vi "Configure Transform Precoding.vi"(6 "Enabled (On)":bool=TRUE, 7 "Bandwidth Part (BWP0)":T1 items=["BWP0"], 8 "error in (no error)":errorcluster, 9 "Carrier Component (1)":T2=1, 10 "Instance (1)":T3=1, 11 "VISA resource name":refnum<visa-resource-name>) -> (0 "error out":errorcluster, 3 "VISA resource name out":refnum<visa-resource-name>)   [LabVIEW 2020, in "Rohde&Schwarz CMXP NR FR2 Measurement.lvlib"]
doc: "Specifies whether the <BWP> on carrier <no> uses a transform precoding function.\n\nAttribute:\nRSCMXPNRFR2M_ATTR_TRANSFORM_PRECODING\n\nRemote-control command:\nCONFigure:NRMMw:MEAS<i>[:CC<no>]:BWPart:PUSCh:DFTPrecoding"
uses:
  <instrlib>/Rohde&Schwarz CMXP NR FR2 Measurement/Rohde&Schwarz CMXP NR FR2 Measurement.lvlib
  <instrlib>/Rohde&Schwarz CMXP NR FR2 Measurement/Private/_Instance.ctl
  <instrlib>/Rohde&Schwarz CMXP NR FR2 Measurement/Private/_Carrier Component.ctl
  <instrlib>/Rohde&Schwarz CMXP NR FR2 Measurement/Private/_Bandwidth Part.ctl
  <instrlib>/Rohde&Schwarz CMXP NR FR2 Measurement/Private/rsidr_core.llb/rsidr_core.lvlib
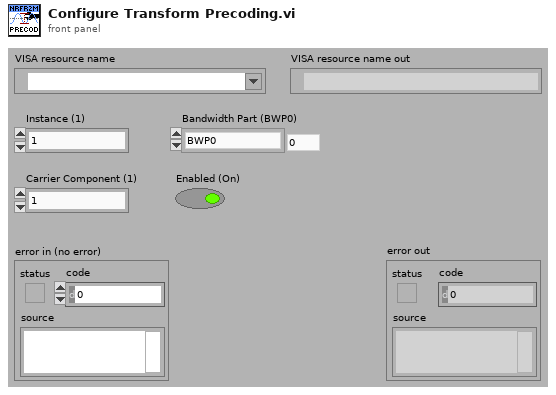
[diagram p1: front panel]
types:
  T1 = typedef "Rohde&Schwarz CMXP NR FR2 Measurement.lvlib/_Bandwidth Part.ctl" = i32
  T2 = typedef "Rohde&Schwarz CMXP NR FR2 Measurement.lvlib/_Carrier Component.ctl" = i32
  T3 = typedef "Rohde&Schwarz CMXP NR FR2 Measurement.lvlib/_Instance.ctl" = i32
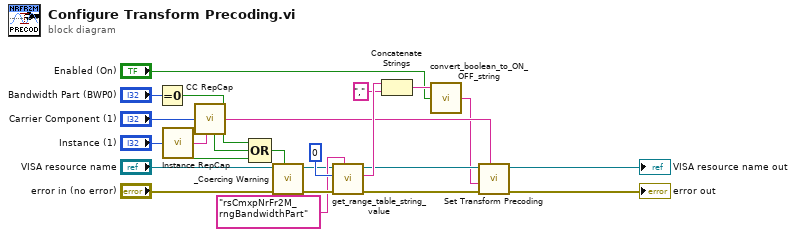
[diagram p0: block diagram]
diagram:
  n1 = Equal To 0?(x="Bandwidth Part (BWP0)") -> (x = 0?=w4:bool)
  n2 = call <instrlib>:"Instance RepCap.vi"("Instance In"="Instance (1)") -> ("In Range?"=w20:bool, "RepCap Identifier Out"=w2:string)  [unwired: 1 in]
  n3 = call <instrlib>:"CC RepCap.vi"("CC In"="Carrier Component (1)", "RepCap String In (\"\")"=w2) -> ("In Range?"=w19:bool, "RepCap Identifier Out"=w11:string)
  n4 = Compound Arithmetic op=OR(w4, w19, w20) -> (w21:bool)
  n5 = call <instrlib>:"_Coercing Warning.vi"("In Range?"=w21, "error in (no error)"="error in (no error)", "VISA resource name"="VISA resource name") -> ("error out"=w17:errorcluster, "VISA resource name out"=w5:refnum<visa-resource-name>)  [unwired: 7 in]
  n6 = call <instrlib>:"get_range_table_string_value.vi"("Range Table ID in"="rsCmxpNrFr2M_rngBandwidthPart", "error in"=w17, "I32 input"=0, "VISA resource name"=w5) -> ("error out"=w10:errorcluster, "String Value out"=w15:string, "VISA resource name out"=w9:refnum<visa-resource-name>)  [unwired: 5 in]
  n7 = Concatenate Strings(w15, "," ("string")) -> (w13:string)
  n8 = call <instrlib>:"convert_boolean_to_ON_OFF_string.vi"("boolean value in"="Enabled (On)", "String to add before (\"\")"=w13) -> ("string value out"=w1:string)  [unwired: 3 in]
  n9 = call "Set Transform Precoding"("Repeated Capabilities"=w11, "error in (no error)"=w10, "Transform Precoding ()"=w1, "instrument handle"=w9) -> ("error out"=→"error out":errorcluster, "instrument handle out"=→"VISA resource name out":refnum<visa-resource-name>)  [unwired: 6 in]
